vi "Save ID Behind Path Recursive.vi"(7 "Paths Dict In":variant, 8 "Error In":errorcluster, 9 "Parent Path":string[](array[string]), 10 "Parent IDs":string[](array[string]), 11 "Tree Dict In":variant) -> (0 "Error Out":errorcluster, 3 "Tree Dict Out":variant, 5 "Paths Dict Out":variant)   [LabVIEW 2020, in "NI_VIAnCFGDataStructure.lvlib" / "Tree.lvclass"]
uses:
  <vilib>/addons/analyzer/VIAnCFGDataStructure/Tree Manager/Tree.lvclass
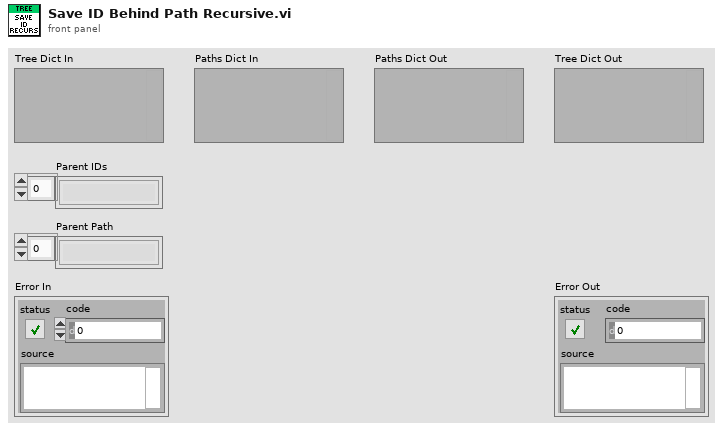
[diagram p1: front panel]
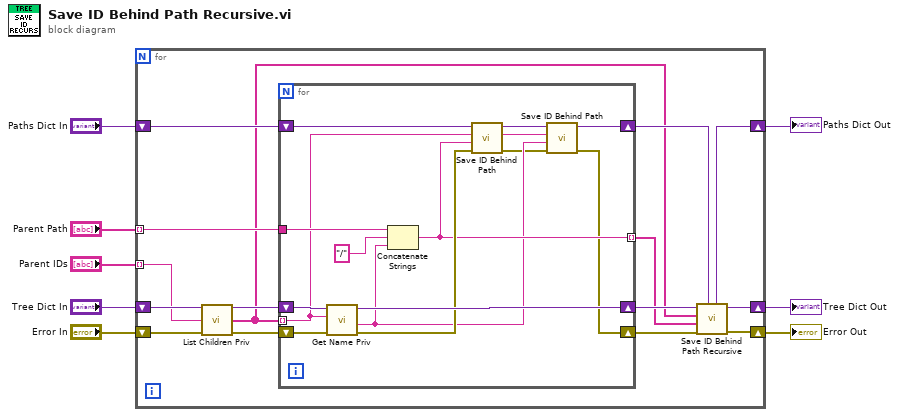
[diagram p0: block diagram]
diagram:
  n1 = for {
    tunnel: "Parent IDs" -> [w14] mode=indexing
    tunnel: "Parent Path" -> [w21] mode=indexing
    shift-right: [w15] -> w7
    shift-left: "Tree Dict In" -> [w23]
    shift-right: [w17] -> w6
    shift-left: "Paths Dict In" -> [w13]
    shift-right: [w16] -> w8
    shift-left: "Error In" -> [w20]
    n2 = call <vilib>:"List Children Priv.vi"("Tree Dictionary"=w23, "Parent ID"=w14, "Error In"=w20) -> ("Tree Dictionary Out"=w22:variant, "Child IDs"=w11:string[], "Error Out"=w19:errorcluster)  [unwired: 10 in]
    n3 = for {
      shift-right: [w36] -> w18
      shift-left: w22 -> [w37]
      tunnel: w11 -> [w28] mode=indexing
      tunnel: w21 -> [w33]
      shift-right: [w24] -> w10
      shift-left: w19 -> [w35]
      shift-right: [w27] -> w12
      shift-left: w13 -> [w32]
      tunnel: [w30] -> w9 mode=indexing
      n4 = call <vilib>:"Get Name Priv.vi"("error in"=w35, "Unique ID"=w28, "Tree Dictionary"=w37) -> ("error out"=w31:errorcluster, "Name"=w26:string, "Tree Dictionary Out"=w36:variant)  [unwired: 6 in]
      n5 = Concatenate Strings(w33, "/" ("string"), w26) -> (w30:string)
      n6 = call <vilib>:"Save ID Behind Path.vi"("Error In"=w31, "Paths"=w30, "IDs"=w28, "Paths Dict"=w32) -> ("Error Out"=w25:errorcluster, "Paths Dict"=w29:variant)  [unwired: 6 in]
      n7 = call <vilib>:"Save ID Behind Path.vi"("Error In"=w25, "Paths"=w26, "IDs"=w28, "Paths Dict"=w29) -> ("Error Out"=w24:errorcluster, "Paths Dict"=w27:variant)  [unwired: 6 in]
    }
    n8 = call <vilib>:"Save ID Behind Path Recursive.vi"("Paths Dict In"=w12, "Error In"=w10, "Parent Path"=w9, "Parent IDs"=w11, "Tree Dict In"=w18) -> ("Error Out"=w16:errorcluster, "Tree Dict Out"=w15:variant, "Paths Dict Out"=w17:variant)  [unwired: 4 in]
  }
  "Error Out" <- w8
  "Tree Dict Out" <- w7
  "Paths Dict Out" <- w6
